vi "BATT-ABSOLUTE.vi"(0 "A4":dbl, 1 "A3":dbl, 2 "A2":dbl, 3 "A1":dbl, 5 "Comp":dbl, 7 "A5":dbl, 9 "B5":dbl, 11 "B1":dbl, 12 "B2":dbl, 13 "B3":dbl, 14 "B4":dbl) -> (4 "Boolean":bool)   [LabVIEW 2016]
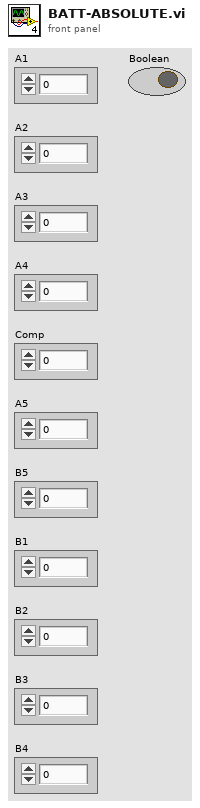
[diagram p1: front panel]
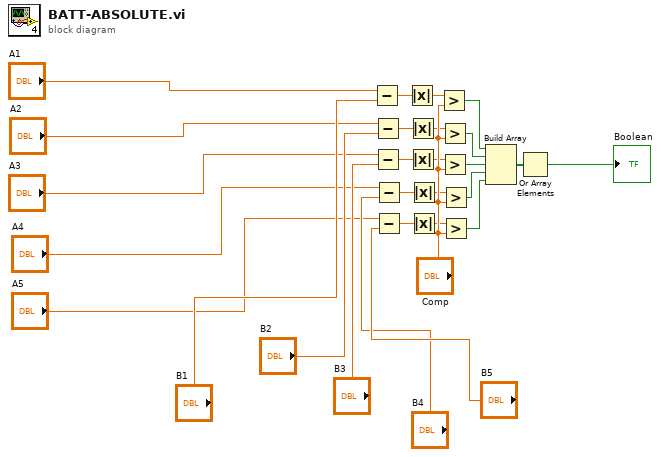
[diagram p0: block diagram]
diagram:
  n1 = Subtract(x="A1", y="B1") -> (x-y=w2:dbl)
  n2 = Subtract(x="A2", y="B2") -> (x-y=w4:dbl)
  n3 = Subtract(x="A3", y="B3") -> (x-y=w6:dbl)
  n4 = Subtract(x="A4", y="B4") -> (x-y=w8:dbl)
  n5 = Subtract(x="A5", y="B5") -> (x-y=w10:dbl)
  n6 = Absolute Value(x=w2) -> (abs(x)=w1:dbl)
  n7 = Absolute Value(x=w4) -> (abs(x)=w3:dbl)
  n8 = Absolute Value(x=w6) -> (abs(x)=w5:dbl)
  n9 = Absolute Value(x=w8) -> (abs(x)=w7:dbl)
  n10 = Absolute Value(x=w10) -> (abs(x)=w9:dbl)
  n11 = Greater?(x=w1, y="Comp") -> (0:w12:bool)
  n12 = Greater?(x=w3, y="Comp") -> (0:w13:bool)
  n13 = Greater?(x=w5, y="Comp") -> (0:w14:bool)
  n14 = Greater?(x=w7, y="Comp") -> (0:w15:bool)
  n15 = Greater?(x=w9, y="Comp") -> (0:w16:bool)
  n16 = Build Array(w12, w13, w14, w15, w16) -> (w17:bool[])
  n17 = Or Array Elements(Boolean array=w17) -> (logical OR=→"Boolean":bool)
